vi "fblue.vi"(7 "LVWS Req":refnum<class "Web Request.lvclass">, 11 "Rate":i32) -> ()   [LabVIEW 2014]
uses:
  <vilib>/wsapi/Web Request.lvclass
  Controller/Controls/Enqueuer Enum.ctl
  CRDS/Actor Messages/Change Laser Rep Rate/Change Laser Rep Rate.lvclass
  CRDS/Actor Messages/Change Laser Rep Rate/Change Laser Rep Rate.lvclass/Change Laser Rep Rate.ctl
  Instr Actor/Messages/Change Blue Laser Rate/Change Blue Laser Rate MSG.lvclass
  Controller/Controller.lvclass
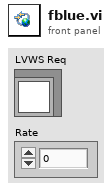
[diagram p1: front panel]
types:
  T1 = typedef "Controller.lvlib/Controller.lvclass/Enqueuer Enum.ctl" = enum8{"PAS", "CRDS", "File", "O3Lamp"}
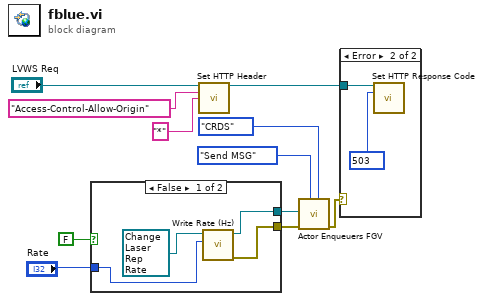
[diagram p0: block diagram]
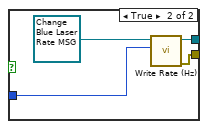
[diagram p2: hidden frame]
diagram:
  n1 = case shown="False" FALSE {
    tunnel: [w13 w18] -> w11
    tunnel: [w12 w17] -> w8
    tunnel: "Rate" -> [w14 w16]
    frame False {
      n2 = call "Write Rate (Hz).vi"("Rate (Hz)"=w14, "Change Laser Rep Rate in"=refnum<class "Change Laser Rep Rate.lvclass"> refnum ("eCRDS Library.lvlib:Change Laser Rep Rate.lvclass")) -> ("error out"=w12:errorcluster, "Change Laser Rep Rate out"=w13:refnum<class "Change Laser Rep Rate.lvclass">)  [unwired: 8 in]
    }
    frame True {
      n3 = call "Write Rate (Hz).vi"("Rate (Hz)"=w16, "Change Blue Laser Rate MSG in"=refnum<class "Change Blue Laser Rate MSG.lvclass"> refnum ("Instrument Lib:Change Blue MSG")) -> ("error out"=w17:errorcluster, "Change Blue Laser Rate MSG out"=w18:refnum<class "Change Blue Laser Rate MSG.lvclass">)  [unwired: 8 in]
    }
  }
  n4 = call <vilib>:"Set HTTP Header.vi"("LabVIEW Web Service Request"="LVWS Req", "header"="Access-Control-Allow-Origin", "header value"="*") -> ("LabVIEW Web Service Request out"=w3:refnum<class "Web Request.lvclass">)  [unwired: 11 in, 1 out]
  n5 = call "Actor Enqueuers FGV.vi"("Enqueuer"=Enqueuer_Enum."CRDS", "State"=enum16{"Store", "Send MSG"}."Send MSG", "error in"=w8, "MSG"=w11) -> ("error out"=w7:errorcluster)  [unwired: 7 in]
  n6 = case shown="Error" w7 {
    tunnel: w3 -> [_ w21]
    frame No Error {
    }
    frame Error {
      w20 = 503 items=["100"=100, "101"=101, "200"=200, "201"=201, "202"=202, "203"=203, "204"=204, "205"=205, "206"=206, "300"=300, "301"=301, "302"=302, "303"=303, "304"=304, "305"=305, "306"=306, "307"=307, "400"=400, "401"=401, "402"=402, "403"=403, "404"=404, "405"=405, "406"=406, "407"=407, "408"=408, "409"=409, "410"=410, "411"=411, "412"=412, "413"=413, "414"=414, "415"=415, "416"=416, "417"=417, "500"=500, "501"=501, "502"=502, "503"=503, "504"=504, "505"=505] ("response code (200)")
      n7 = call <vilib>:"Set HTTP Response Code.vi"("LabVIEW Web Service Request"=w21, "response code (200)"=w20) -> ()  [unwired: 12 in, 2 out]
    }
  }
